vi "Test - Init Definitions.vi"   [LabVIEW 2020, in "JSON Schema Generator.lvlib"]
uses:
  JSON Schema Generator.lvlib
  <vilib>/addons/_JKI Toolkits/Caraya/classes/Test/Test.lvclass
  <vilib>/addons/_JKI Toolkits/Caraya/classes/Assert/Assert.lvclass
  <vilib>/addons/_JKI Toolkits/Caraya/classes/Assert/Assert Equal Value_Variant.vi
  <vilib>/addons/_JKI Toolkits/Caraya/classes/Assert/Assert Not Error.vi
  Defintion FGV Actions.ctl
types:
  T1 = typedef "JSON Schema Generator.lvlib/Defintion FGV Actions.ctl" = enum16{"Create Defs", "Update Defs", "Get all Defs", "Get Def"}
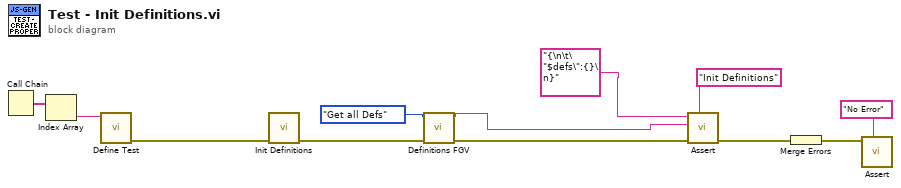
[diagram p0: block diagram]
diagram:
  n1 = Call Chain() -> (call chain=w12:string[])
  n2 = Index Array(array=w12) -> (element=w11:string)  [unwired: 1 in]
  n3 = call <vilib>:"Define Test.vi"("Label (VI Title)"=w11) -> ("error out"=w6:errorcluster)  [unwired: 9 in, 1 out]
  n4 = call "Init Definitions.vi"("error in (no error)"=w6) -> ("error out (no error)"=w4:errorcluster)  [unwired: 10 in]
  n5 = call "Definitions FGV.vi"("error in (no error)"=w4, "Action"=Defintion_FGV_Actions."Get all Defs") -> ("error out"=w3:errorcluster, "Definitions out"=w1:string)  [unwired: 7 in, 1 out]
  n6 = call-poly <vilib>:"Assert.vi"("Label"="Init Definitions", "error in (no error)"=w3, "Actual"=w1, "Expected"="{\n\t\"$defs\":{}\n}") -> ("error out"=w9:errorcluster)  [unwired: 6 in, 1 out]
  n7 = Merge Errors(w9) -> (w7:errorcluster)
  n8 = call-poly <vilib>:"Assert.vi"("Label"="No Error", "Not Error?"=w7) -> ()  [unwired: 8 in, 2 out]
